vi "Get Text.vi"(8 "error in (no error)":errorcluster, 11 "Text In":refnum<class "Text.lvclass">) -> (0 "error out":errorcluster, 2 "Text":string, 3 "Text Out":refnum<class "Text.lvclass">)   [LabVIEW 2017, in "Front Panel Publisher.lvlib" / "Text.lvclass"]
uses:
  Text.lvclass
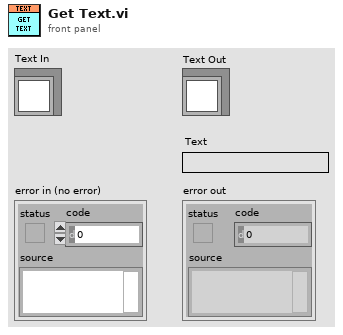
[diagram p1: front panel]
types:
  T1 = typedef "Front Panel Publisher.lvlib/Text.lvclass/Attributes.ctl" = cluster{"Text":string, "Font":string, "Font Size":u32, "Visible":bool, "Control Reference":refnum<vi>}
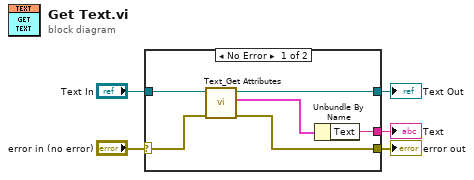
[diagram p0: block diagram]
diagram:
  n1 = case shown="No Error" "error in (no error)" {
    selector: "error in (no error)" -> [w11 w13]
    tunnel: [w9 w13] -> w4
    tunnel: [w7 w12] -> w2
    tunnel: "Text In" -> [w8 w12]
    tunnel: [w6 _] -> w1
    frame No Error {
      n2 = call "Text_Get Attributes.vi"("error in (no error)"=w11, "Text In"=w8) -> ("error out"=w9:errorcluster, "Data"=w10:T1, "Text Out"=w7:refnum<class "Text.lvclass">)  [unwired: 7 in]
      n3 = Unbundle By Name(w10) -> ("Text"=w6:string)
    }
    frame Error {
    }
  }
  "error out" <- w4
  "Text Out" <- w2
  "Text" <- w1
